vi "E3631A_Voltage Controller.vi"(0 "VISA resource name":refnum<visa-resource-name>="GPIB0::5::INSTR", 1 "I_VDD(A)":dbl=0.2 format="%.3g", 2 "Initialize":bool, 3 "Channel Controller":T1(ring)=enum."Voltage 3", 5 "Voltage 1":dbl=3.3 format="%.3g", 9 "Voltage 2":dbl=3.3 format="%.3g", 11 "error in (no error)":errorcluster, 12 "Voltage 3":dbl=-3.3 format="%.3g", 13 "I_3.3V (A)":dbl=0.2 format="%.3g", 14 "I_-3.3V(A)":dbl format="%.3g") -> (4 "VISA resource name out":refnum<visa-resource-name>="GPIB0::5::INSTR", 15 "error out":errorcluster)   [LabVIEW 2012]
uses:
  Agilent E363X Series/Agilent E363X Series.lvlib
panel:
  in  "Channel 3":i32(ring)=3 items=["Channel 1"=1, "Channel 2"=2, "Channel 3"=3]
  in  "Channel 2":i32(ring)=2 items=["Channel 1"=1, "Channel 2"=2, "Channel 3"=3]
  in  "Channel 1":i32(ring)=1 items=["Channel 1"=1, "Channel 2"=2, "Channel 3"=3]
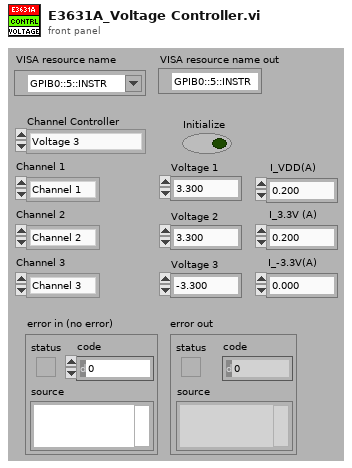
[diagram p1: front panel]
types:
  T1 = enum16{"Idle...", "Voltage 1", "Voltage 2", "Voltage 3"}
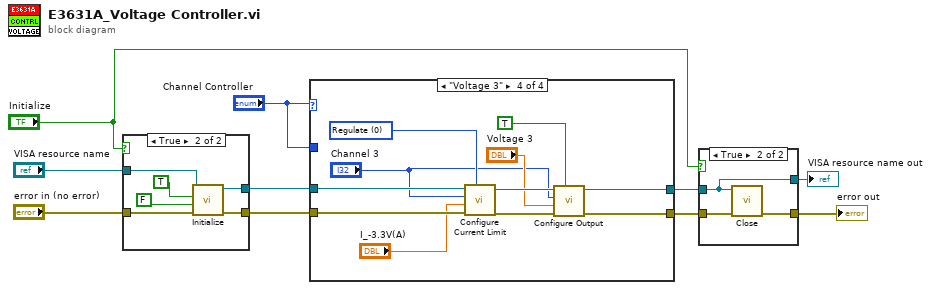
[diagram p0: block diagram]
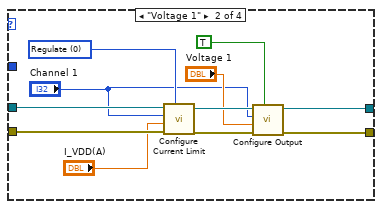
[diagram p5: hidden frame]
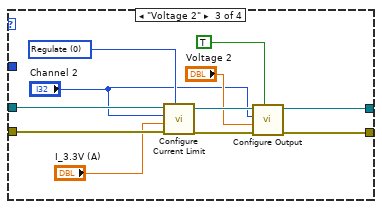
[diagram p6: hidden frame]
diagram:
  n1 = case shown="True" "Initialize" {
    tunnel: "error in (no error)" -> [w11 w18]
    tunnel: [w11 w17] -> w9
    tunnel: [w12 w16] -> w8
    tunnel: "VISA resource name" -> [w12 w13]
    frame False {
    }
    frame True {
      n2 = call "Initialize.vi"("error in (no error)"=w18, "Reset? (T: Yes)"=FALSE, "ID Query? (T: Yes)"=TRUE, "VISA resource name"=w13) -> ("error out"=w17:errorcluster, "VISA resource name out"=w16:refnum<visa-resource-name>)  [unwired: 6 in]
    }
  }
  n3 = case shown="\"Voltage 3\"" "Channel Controller" {
    tunnel: w9 -> [w19 w31 w42 w53]
    tunnel: w8 -> [w20 w30 w41 w52]
    tunnel: [w19 w25 w36 w47] -> w7
    tunnel: [w20 w24 w35 w46] -> w6
    tunnel: "Channel Controller" -> [_ _ _ _]
    frame "Idle...", Default {
    }
    frame "Voltage 1" {
      w29 = u16 0 items=["Regulate", "Trip"] ("Behavior (0: Regulate)")
      n4 = call "Configure Current Limit.vi"("Behavior (0: Regulate)"=w29, "error in (no error)"=w31, "Current Limit (0.0 A)"="I_VDD(A)", "Channel (1: Channel 1)"="Channel 1", "VISA resource name"=w30) -> ("error out"=w27:errorcluster, "VISA resource name out"=w28:refnum<visa-resource-name>)  [unwired: 5 in]
      n5 = call "Configure Output.vi"("Enable Output (T: Enable)"=TRUE, "error in (no error)"=w27, "Voltage Level (0.0 V)"="Voltage 1", "Channel (1: Channel 1)"="Channel 1", "VISA resource name"=w28) -> ("error out"=w25:errorcluster, "VISA resource name out"=w24:refnum<visa-resource-name>)  [unwired: 5 in]
    }
    frame "Voltage 2" {
      w40 = u16 0 items=["Regulate", "Trip"] ("Behavior (0: Regulate)")
      n6 = call "Configure Current Limit.vi"("Behavior (0: Regulate)"=w40, "error in (no error)"=w42, "Current Limit (0.0 A)"="I_3.3V (A)", "Channel (1: Channel 1)"="Channel 2", "VISA resource name"=w41) -> ("error out"=w38:errorcluster, "VISA resource name out"=w39:refnum<visa-resource-name>)  [unwired: 5 in]
      n7 = call "Configure Output.vi"("Enable Output (T: Enable)"=TRUE, "error in (no error)"=w38, "Voltage Level (0.0 V)"="Voltage 2", "Channel (1: Channel 1)"="Channel 2", "VISA resource name"=w39) -> ("error out"=w36:errorcluster, "VISA resource name out"=w35:refnum<visa-resource-name>)  [unwired: 5 in]
    }
    frame "Voltage 3" {
      w51 = u16 0 items=["Regulate", "Trip"] ("Behavior (0: Regulate)")
      n8 = call "Configure Current Limit.vi"("Behavior (0: Regulate)"=w51, "error in (no error)"=w53, "Current Limit (0.0 A)"="I_-3.3V(A)", "Channel (1: Channel 1)"="Channel 3", "VISA resource name"=w52) -> ("error out"=w49:errorcluster, "VISA resource name out"=w50:refnum<visa-resource-name>)  [unwired: 5 in]
      n9 = call "Configure Output.vi"("Enable Output (T: Enable)"=TRUE, "error in (no error)"=w49, "Voltage Level (0.0 V)"="Voltage 3", "Channel (1: Channel 1)"="Channel 3", "VISA resource name"=w50) -> ("error out"=w47:errorcluster, "VISA resource name out"=w46:refnum<visa-resource-name>)  [unwired: 5 in]
    }
  }
  n10 = case shown="True" "Initialize" {
    tunnel: w7 -> [w55 w58]
    tunnel: w6 -> [w54 w56]
    tunnel: [w55 w57] -> w5
    tunnel: [w54 w56] -> w1
    frame False {
    }
    frame True {
      n11 = call "Close.vi"("error in (no error)"=w58, "VISA resource name"=w56) -> ("error out"=w57:errorcluster)  [unwired: 9 in]
    }
  }
  "error out" <- w5
  "VISA resource name out" <- w1
